vi "FTW-Connector-SpawnNewActor.vi"(0 "Instance Configuration":string="{\n  \"Identity\": \"ActorName\",\n  \"InboxAddress\": \"tcp://127.0.0.1:*\",\n  \"HandshakeTimeout\": 1000,\n  \"DebugEnableInboxLogging\": false,\n  \"DebugEnableJobLogging\": false,\n  \"DebugShowPanel\": false\n}", 2 "FTW Actor Connector Type":refnum<class "FTW-Actor-Connector.lvclass">, 11 "error in":errorcluster) -> (4 "FTW Actor Connector":refnum<class "FTW-Actor-Connector.lvclass">, 6 "Instance Inbox Address":string, 8 "Instance VI Clone Name":string, 15 "error out":errorcluster)   [LabVIEW 2014, in "FTW-Actor-Connector.lvclass"]
uses:
  FTW-Actor-Connector.lvclass
  lib/FTW-LibraryFilepath.vi
  reflection/FTW-Reflection-Type.vi
  error/FTW-ERR-StatusException.vi
  error/FTW-ERR-ThrowGenericError.vi
  error/FTW-ERR-ThrowError.vi
  error/FTW-ERR-NoErrorConstant.vi
  json/FTW-JSON-Construct-FromBuffer.vi
  error/FTW-ERR-CallChain.vi
  string/FTW-STR-ReplaceWhitespace.vi
  reflection/FTW-Reflection-Array.vi
  json/core/FTW-JSON-Core-GetFlattenedValue.vi
  json/FTW-JSON-Destroy.vi
  json/FTW-JSON-Deserialize/FTW-JSON-Deserialize.xnode
panel:
  # "Inputs"
  # "Outputs"
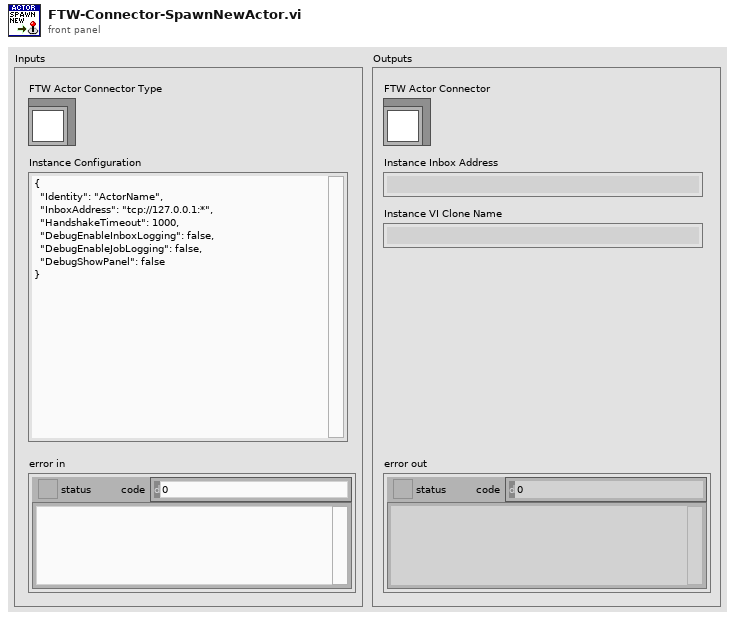
[diagram p1: front panel]
types:
  T1 = cluster{"FTW-PrimaryInboxAddress":string, "FTW-InstanceCloneName":string}
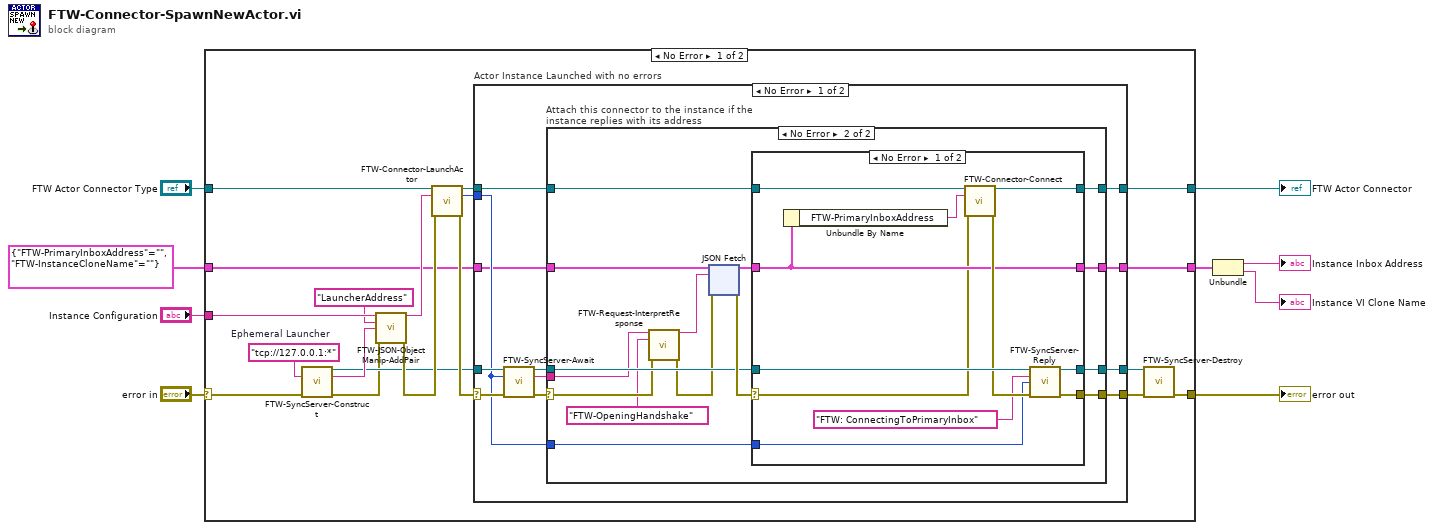
[diagram p0: block diagram]
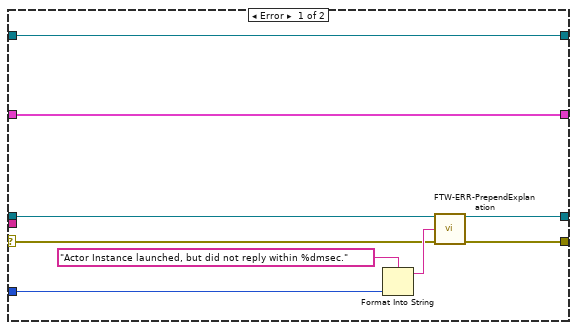
[diagram p2: hidden frame]
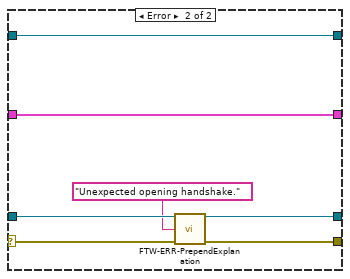
[diagram p3: hidden frame]
diagram:
  n1 = case shown="No Error" "error in" {
    selector: "error in" -> [w13 w119]
    tunnel: [w23 w119] -> w5
    tunnel: [w28 w118] -> w6
    tunnel: "FTW Actor Connector Type" -> [w22 w118]
    tunnel: "Instance Configuration" -> [w27 _]
    tunnel: T1 {"FTW-PrimaryInboxAddress"="", "FTW-InstanceCloneName"=""} -> [w11 w117]
    tunnel: [w10 w117] -> w3
    frame No Error {
      w16 = "tcp://127.0.0.1:*"  # Ephemeral Launcher
      n2 = call "FTW-SyncServer-Construct.vi"("Instance Inbox Address"=w16, "error in"=w13) -> ("FTW Synchronous Server"=w14:refnum<data-value>, "Resolved Inbox Address"=w15:string, "error out"=w12:errorcluster)  [unwired: 11 in]
      n3 = call "FTW-JSON-ObjectManip-AddPair.vi"("Input JSON Object"=w27, "Key"="LauncherAddress", "Value"=w15, "error in"=w12) -> ("Output JSON Object"=w18:string, "error out"=w20:errorcluster)  [unwired: 10 in]
      n4 = call-dynamic "FTW-Connector-LaunchActor.vi"("FTW Actor Connector"=w22, "Actor Instance Configuration"=w18, "error in"=w20) -> ("FTW Actor Connector out"=w21:refnum<class "FTW-Actor-Connector.lvclass">, "Handshake Timeout"=w17:i32, "error out"=w19:errorcluster)  [unwired: 10 in]
      n5 = case "Actor Instance Launched with no errors" shown="No Error" w19 {
        selector: w19 -> [w34 w115]
        tunnel: [w40 w115] -> w24
        tunnel: w21 -> [w39 w116]
        tunnel: [w38 w116] -> w28
        tunnel: w14 -> [w36 w114]
        tunnel: [w37 w114] -> w25
        tunnel: [w29 w113] -> w10
        tunnel: w17 -> [w32 _]
        tunnel: w11 -> [w30 w113]
        frame No Error {
          n6 = call "FTW-SyncServer-Await.vi"("FTW Synchronous Server"=w36, "Receive Timeout"=w32, "error in"=w34) -> ("FTW Synchronous Server out"=w35:refnum<data-value>, "Incoming Request"=w31:string, "error out"=w33:errorcluster)  [unwired: 10 in]
          n7 = case "Attach this connector to the instance if the instance replies with its address" shown="No Error" w33 {
            selector: w33 -> [w42 w53]
            tunnel: [w41 w61] -> w40
            tunnel: w39 -> [w48 w63]
            tunnel: [w48 w62] -> w38
            tunnel: w35 -> [w47 w55]
            tunnel: [w47 w56] -> w37
            tunnel: w32 -> [w45 w60]
            tunnel: w31 -> [_ w51]
            tunnel: w30 -> [w44 w58]
            tunnel: [w44 w54] -> w29
            frame Error {
              n8 = Format Into String(format string="Actor Instance launched, but did not reply within %dmsec." ("Error Message"), w45) -> (resulting string=w43:string)  [unwired: 2 in, 1 out]
              n9 = call "FTW-ERR-PrependExplanation.vi"("Exception Information"=w43, "error in"=w42) -> ("error out"=w41:errorcluster)  [unwired: 13 in]
            }
            frame No Error {
              n10 = call "FTW-Request-InterpretResponse.vi"("Raw Request"=w51, "Request Header"="FTW-OpeningHandshake", "error in"=w53) -> ("JSON Response"=w50:string, "error out"=w52:errorcluster)  [unwired: 11 in]
              n11 = xnode "JSON Fetch"("Type and Defaults"=w58, "JSON String"=w50, "error in"=w52) -> ("Values"=w57:T1, "error out"=w59:errorcluster)  [unwired: 1 in]
              n12 = case shown="No Error" w59 {
                selector: w59 -> [w98 w108]
                tunnel: w63 -> [w106 w112]
                tunnel: [w105 w112] -> w62
                tunnel: [w96 w111] -> w61
                tunnel: w57 -> [w100 w109]
                tunnel: w55 -> [w103 w110]
                tunnel: w60 -> [w99 _]
                tunnel: [w97 w110] -> w56
                tunnel: [w100 w109] -> w54
                frame No Error {
                  n13 = Unbundle By Name(w100) -> ("FTW-PrimaryInboxAddress"=w104:string)
                  n14 = call "FTW-Connector-Connect.vi"("FTW Actor Connector"=w106, "Instance Inbox Address"=w104, "error in"=w98) -> ("FTW Actor Connector out"=w105:refnum<class "FTW-Actor-Connector.lvclass">, "error out"=w102:errorcluster)  [unwired: 11 in]
                  n15 = call "FTW-SyncServer-Reply.vi"("FTW Synchronous Server"=w103, "Response"="FTW: ConnectingToPrimaryInbox" ("Message Header"), "Send Timeout"=w99, "error in"=w102) -> ("FTW Synchronous Server out"=w97:refnum<data-value>, "error out"=w96:errorcluster)  [unwired: 10 in]
                }
                frame Error {
                  n16 = call "FTW-ERR-PrependExplanation.vi"("Exception Information"="Unexpected opening handshake.", "error in"=w108) -> ("error out"=w111:errorcluster)  [unwired: 13 in]
                }
              }
            }
          }
        }
        frame Error {
        }
      }
      n17 = call "FTW-SyncServer-Destroy.vi"("FTW Synchronous Server"=w25, "error in"=w24) -> ("error out"=w23:errorcluster)  [unwired: 13 in]
    }
    frame Error {
    }
  }
  "error out" <- w5
  "FTW Actor Connector" <- w6
  n18 = Unbundle(w3) -> ("FTW-PrimaryInboxAddress"=→"Instance Inbox Address":string, "FTW-InstanceCloneName"=→"Instance VI Clone Name":string)
